vi "Create FPGA Target.vi"(10 "target class":string, 11 "Parent Item In":refnum<vi>) -> (3 "target structure name":string)   [LabVIEW 2020, in "NI_TargetHelper.lvlib"]
uses:
  <vilib>/TargetSupport/NI_TargetHelper/NI_TargetHelper.lvlib
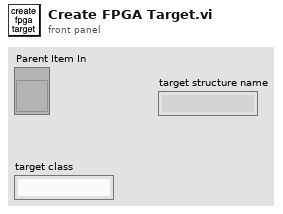
[diagram p1: front panel]
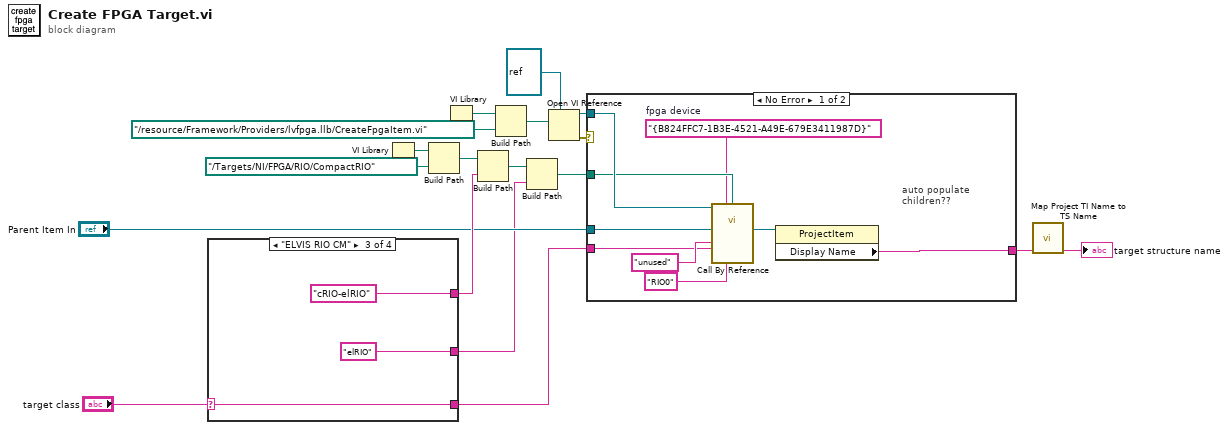
[diagram p0: block diagram]
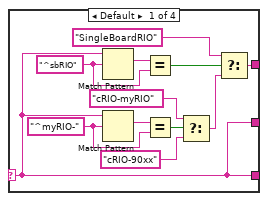
[diagram p2: hidden frame]
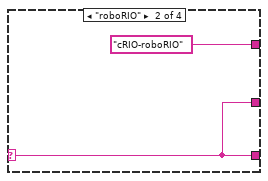
[diagram p3: hidden frame]
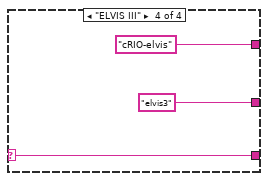
[diagram p4: hidden frame]
diagram:
  n1 = case shown="\"ELVIS RIO CM\"" "target class" {
    selector: "target class" -> [w19 w31 w33 w36]
    tunnel: [w26 "cRIO-roboRIO" "cRIO-elRIO" "cRIO-elvis"] -> w11
    tunnel: [w19 w31 w33 w36] -> w2
    tunnel: [w19 w31 "elRIO" "elvis3"] -> w1
    frame Default {
      w25 = "^myRIO-" ("regular expression")
      w29 = "^sbRIO" ("regular expression")
      n2 = Match Pattern(string=w19, regular expression=w29) -> (match substring=w30:string)  [unwired: 1 in, 3 out]
      n3 = Match Pattern(string=w19, regular expression=w25) -> (match substring=w24:string)  [unwired: 1 in, 3 out]
      n4 = Equal?(x=w30, y=w29) -> (x = y?=w28:bool)
      n5 = Equal?(x=w24, y=w25) -> (x = y?=w23:bool)
      n6 = Select(t="cRIO-myRIO" ("regular expression"), s=w23, f="cRIO-90xx") -> (s? t:f=w21:string)
      n7 = Select(t="SingleBoardRIO" ("regular expression"), s=w28, f=w21) -> (s? t:f=w26:string)
    }
    frame "roboRIO" {
    }
    frame "ELVIS RIO CM" {
    }
    frame "ELVIS III" {
    }
  }
  n8 = VI Library() -> (path=w13:path)
  n9 = Build Path(base path=w13, name or relative path=path "../Targets/NI/FPGA/RIO/CompactRIO") -> (appended path=w14:path)
  n10 = VI Library() -> (path=w4:path)
  n11 = Build Path(base path=w14, name or relative path=w11) -> (appended path=w12:path)
  n12 = Build Path(base path=w4, name or relative path=path "../resource/Framework/Providers/lvfpga.llb/CreateFpgaItem.vi") -> (appended path=w5:path)
  n13 = Build Path(base path=w12, name or relative path=w1) -> (appended path=w7:path)
  n14 = Open VI Reference(type specifier VI Refnum (for type only)=refnum<vi> refnum, vi path=w5) -> (vi reference=w10:refnum<vi>, error out=w9:errorcluster)  [unwired: 4 in]
  n15 = case shown="No Error" w9 {
    tunnel: w10 -> [w47 _]
    tunnel: w2 -> [w45 _]
    tunnel: [w42 _] -> w8
    tunnel: w7 -> [w41 _]
    tunnel: "Parent Item In" -> [w40 _]
    frame No Error {
      w39 = "{B824FFC7-1B3E-4521-A49E-679E3411987D}"  # fpga device
      # "auto populate\nchildren??"
      n16 = call-by-ref "?"(reference=w47, "Parent Item In"=w40, "Item Type"=w39, "Target Path"=w41, "Model Name (UNUSED)"="unused", "Target Class"=w45, "Resource Name (relative)"="RIO0") -> ("Created Item"=w43:refnum<vi>)  [unwired: 8 in, 4 out]
      n17 = property class="ProjectItem"(reference=w43) -> ("Display Name"=w42:string)  [unwired: 1 in, 2 out]
    }
    frame Error {
    }
  }
  n18 = call <vilib>:"Map Project TI Name to TS Name.vi"("project targetitem name"=w8) -> ("target structure name"=→"target structure name":string)  [unwired: 10 in]
